vi "p2.vi"() -> ()   [LabVIEW 2021, in "d18.lvlib"]
uses:
  d18.lvlib
  <vilib>/Math Plots/3D Math Plots/3D Scatter/3D Scatter XCtrl/3D Scatter.xctl
  <vilib>/Math Plots/3D Math Plots/3D Scatter/3D Scatter Datatype/Public/Plot Helper (Vector).vi
  AOC/AOC.lvlib
  <vilib>/Math Plots/3D Math Plots/3D Scatter/3D Scatter Datatype/3D Scatter Datatype.lvclass
panel:
  out "3D Scatter":refnum<class "3D Plot Datatype.lvclass">[](xcontrol)
  in  "Example":string="2,2,2\n1,2,2\n3,2,2\n2,1,2\n2,3,2\n2,2,1\n2,2,3\n2,2,4\n2,2,6\n1,2,5\n3,2,5\n2,1,5\n2,3,5"
  in  "Example":bool=TRUE
  out "Answer":i64
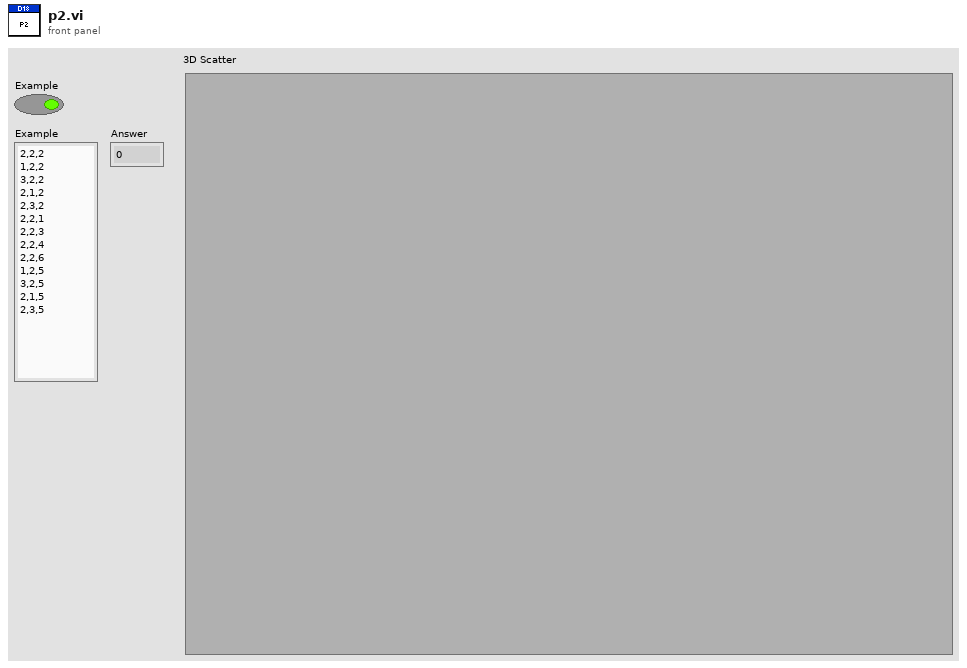
[diagram p1: front panel]
types:
  T1 = cluster{"point":cluster{i64, i64, i64}, "Response Notifier":refnum<notifier>}
  T2 = cluster{cluster{"Point to Set":cluster{i64, i64, i64}, "Internal?":bool}, "notifier out":refnum<notifier>}
  T3 = map{cluster{i64, i64, i64}, cluster{"Set?":bool, "Internal?":bool}}
  T4 = cluster{"key not found?":bool, cluster{"Set?":bool, "Internal?":bool}}
  T5 = cluster{"Point to Set":cluster{i64, i64, i64}, "Internal?":bool}
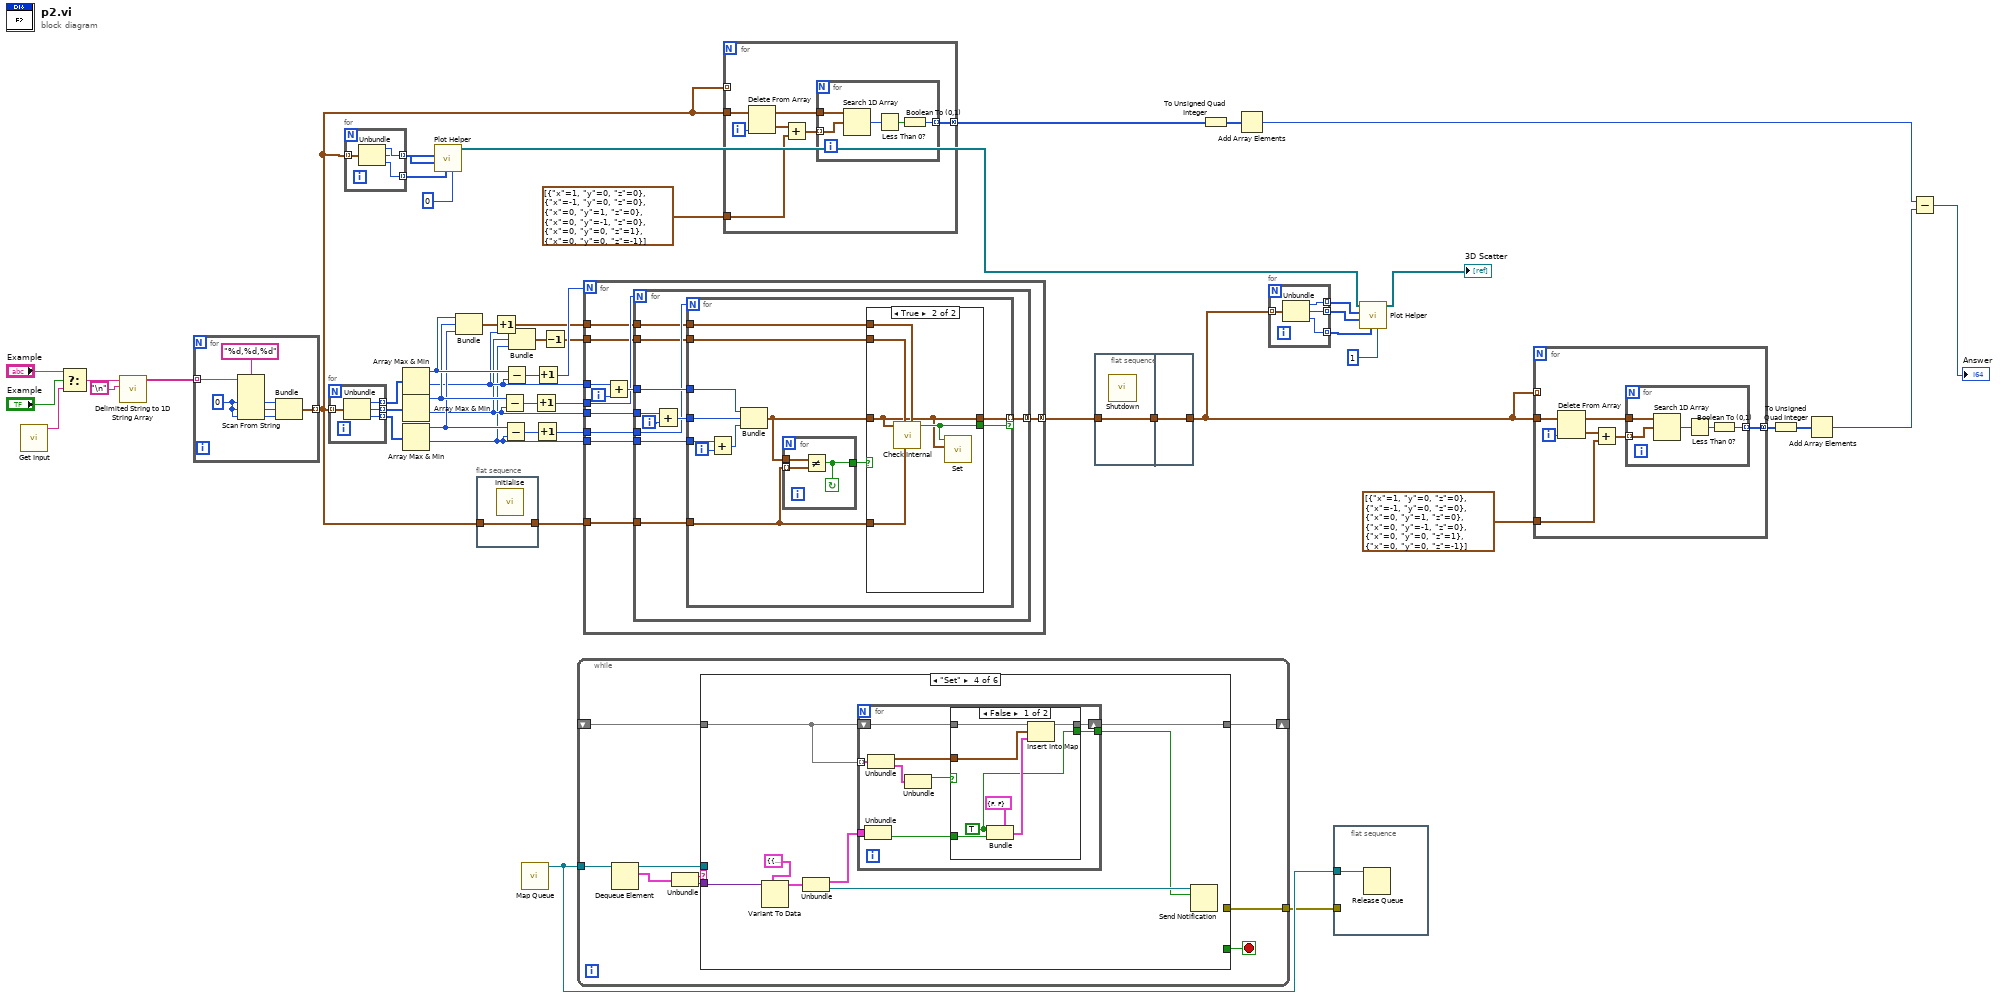
[diagram p0: block diagram]
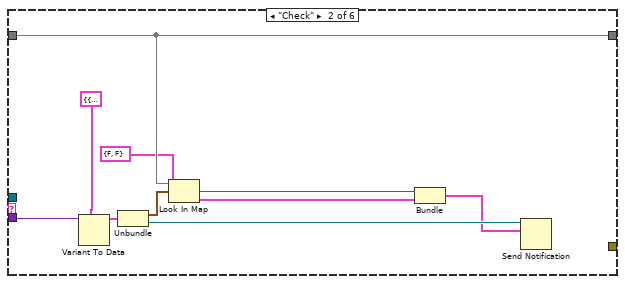
[diagram p3: hidden frame]
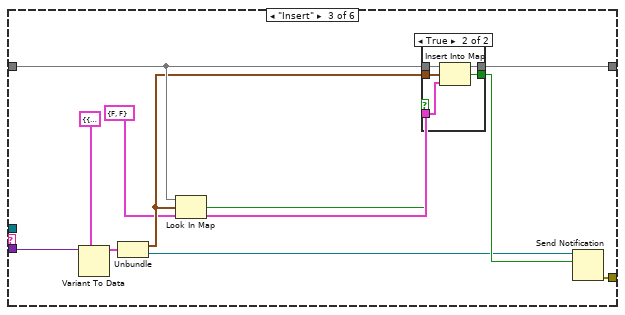
[diagram p4: hidden frame]
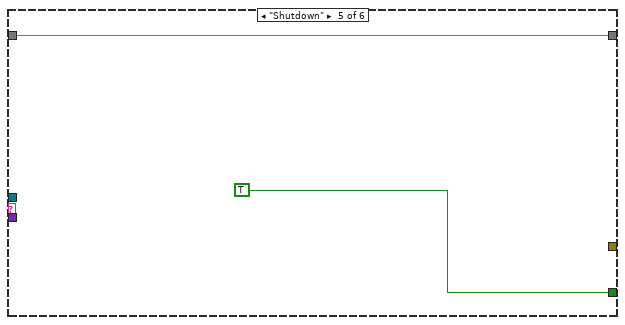
[diagram p7: hidden frame]
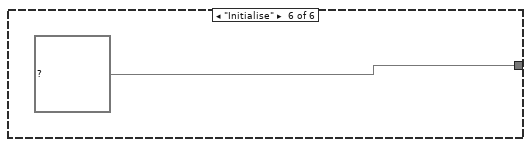
[diagram p8: hidden frame]
diagram:
  n1 = call "Get Input.vi"() -> ("Input"=w51:string)  [unwired: 11 in]
  n2 = Select(t="Example", s="Example", f=w51) -> (s? t:f=w50:string)
  n3 = call <vilib>:"Delimited String to 1D String Array.vi"("delimiter"="\n", "delimited string"=w50) -> ("string array"=w46:string[])  [unwired: 9 in]
  n4 = for {
    tunnel: w46 -> [w58] mode=indexing
    tunnel: [w52] -> w14 mode=indexing
    w56 = i64 0
    n5 = Scan From String(format string="%d,%d,%d", input string=w58, default 1=w56, default 2=w56, default 3=w56) -> (output 1=w55:i64, output 2=w54:i64, output 3=w53:i64)  [unwired: 2 in, 3 out]
    n6 = Bundle(w55, w54, w53) -> (w52:cluster{i64, i64, i64})  [unwired: 1 in]
  }
  n7 = for {
    tunnel: w14 -> [w62] mode=indexing
    tunnel: [w61] -> w45 mode=indexing
    tunnel: [w60] -> w44 mode=indexing
    tunnel: [w59] -> w43 mode=indexing
    n8 = Unbundle(w62) -> (w61:i64, w60:i64, w59:i64)
  }
  n9 = for {
    tunnel: w14 -> [w66] mode=indexing
    tunnel: [w65] -> w13 mode=indexing
    tunnel: [w64] -> w12 mode=indexing
    tunnel: [w63] -> w11 mode=indexing
    n10 = Unbundle(w66) -> (w65:i64, w64:i64, w63:i64)
  }
  n11 = Array Max & Min(array=w45) -> (max value=w36:i64, min value=w33:i64)  [unwired: 2 out]
  n12 = Array Max & Min(array=w44) -> (max value=w35:i64, min value=w32:i64)  [unwired: 2 out]
  n13 = Array Max & Min(array=w43) -> (max value=w34:i64, min value=w31:i64)  [unwired: 2 out]
  n14 = call-poly <vilib>:"Plot Helper.vi"("Plot ID"=0, "z vector"=w11, "y vector"=w12, "x vector"=w13) -> ("3D Plot lvclass Array out"=w9:refnum<class "3D Plot Datatype.lvclass">[])  [unwired: 2 in, 5 out]
  n15 = Bundle(w36, w35, w34) -> (w30:cluster{i64, i64, i64})  [unwired: 1 in]
  n16 = flat-sequence {
    tunnel: w14 -> [w67]
    tunnel: [w67] -> w18
    frame #0 {
      n17 = call "Initialise.vi"() -> ()  [unwired: 12 in]
    }
  }
  n18 = Increment(x=w30) -> (x+1=w2:cluster{i64, i64, i64})
  n19 = Subtract(x=w35, y=w32) -> (x-y=w41:i64)
  n20 = Subtract(x=w34, y=w31) -> (x-y=w39:i64)
  n21 = Subtract(x=w36, y=w33) -> (x-y=w42:i64)
  n22 = Bundle(w33, w32, w31) -> (w29:cluster{i64, i64, i64})  [unwired: 1 in]
  n23 = call "Map Queue.vi"() -> ("Queue out"=w16:refnum<queue>)  [unwired: 11 in]
  n24 = Increment(x=w41) -> (x+1=w40:i64)
  n25 = Increment(x=w39) -> (x+1=w38:i64)
  n26 = Increment(x=w42) -> (x+1=w37:i64)
  n27 = Decrement(x=w29) -> (x-1=w1:cluster{i64, i64, i64})
  n28 = while {
    tunnel: w16 -> [w76]
    shift-right: [w71] -> _
    shift-left: _ -> [w70]
    tunnel: [w68] -> w15
    stop <- w69 stop-if-true
    n29 = Dequeue Element(queue=w76) -> (queue out=w75:refnum<queue>, element=w74:cluster{"Instruction":string, "Data":variant})  [unwired: 2 in, 2 out]
    n30 = Unbundle(w74) -> ("Instruction"=w73:string, "Data"=w72:variant)
    n31 = case shown="\"Set\"" w73 {
      tunnel: w75 -> [_ _ _ _ _ _]
      tunnel: w72 -> [_ w87 w99 w113 _ _]
      tunnel: [w77 w86 w97 w111 w133 T3 {} ("map in")] -> w71
      tunnel: w70 -> [w77 w86 w95 w106 w133 _]
      tunnel: [_ _ _ _ TRUE _] -> w69
      tunnel: [_ _ w88 _ _ _] -> w68
      frame Default {
      }
      frame "Check" {
        n32 = Variant To Data(type=T1 {"point"={0, 0, 0}, "Response Notifier"=refnum}, Variant=w87) -> (data=w85:T1)  [unwired: 1 in, 1 out]
        n33 = Unbundle(w85) -> ("point"=w84:cluster{i64, i64, i64}, "Response Notifier"=w83:refnum<notifier>)
        n34 = Look In Map(map=w86, key=w84, default value=cluster{"Set?":bool, "Internal?":bool} {"Set?"=FALSE, "Internal?"=FALSE}) -> (key not found?=w82:bool, value=w81:cluster{"Set?":bool, "Internal?":bool})
        n35 = Bundle("key not found?"=w82, w81) -> (w80:T4)  [unwired: 1 in]
        n36 = Send Notification(notification=w80, notifier=w83) -> ()  [unwired: 1 in, 2 out]
      }
      frame "Insert" {
        n37 = Variant To Data(type=T1 {"point"={0, 0, 0}, "Response Notifier"=refnum}, Variant=w99) -> (data=w98:T1)  [unwired: 1 in, 1 out]
        n38 = Unbundle(w98) -> ("point"=w94:cluster{i64, i64, i64}, "Response Notifier"=w89:refnum<notifier>)
        n39 = Look In Map(map=w95, key=w94, default value=cluster{"Set?":bool, "Internal?":bool} {"Set?"=FALSE, "Internal?"=FALSE}) -> (key not found?=w91:bool, value=w93:cluster{"Set?":bool, "Internal?":bool})
        n40 = case shown="True" w91 {
          tunnel: [w100 w105] -> w97
          tunnel: [_ w104] -> w96
          tunnel: w95 -> [w100 w103]
          tunnel: w94 -> [_ w102]
          tunnel: w93 -> [_ w101]
          frame False {
          }
          frame True {
            n41 = Insert Into Map(map in=w103, key=w102, value=w101) -> (map out=w105:T3, key already included?=w104:bool)  [unwired: 1 out]
          }
        }
        n42 = Send Notification(notification=w96, notifier=w89) -> (error out=w88:errorcluster)  [unwired: 1 in, 1 out]
      }
      frame "Set" {
        n43 = Variant To Data(type=T2 {{"Point to Set"={0, 0, 0}, "Internal?"=FALSE}, "notifier out"=refnum} ("output cluster"), Variant=w113) -> (data=w112:T2)  [unwired: 1 in, 1 out]
        n44 = Unbundle(w112) -> (w109:T5, "notifier out"=w108:refnum<notifier>)
        n45 = for {
          tunnel: w109 -> [w120]
          tunnel: [w119] -> w107
          shift-right: [w122] -> w111
          shift-left: w106 -> [w121]
          tunnel: w106 -> [w117] mode=indexing
          n46 = Unbundle(w120) -> ("Internal?"=w118:bool)  [unwired: 1 out]
          n47 = Unbundle(w117) -> ("point"=w116:cluster{i64, i64, i64}, "info"=w115:cluster{"Set?":bool, "Internal?":bool})
          n48 = Unbundle(w115) -> ("Set?"=w114:bool)  [unwired: 1 out]
          n49 = case shown="False" w114 {
            tunnel: [w129 w131] -> w122
            tunnel: w121 -> [w128 w131]
            tunnel: [w123 w130] -> w119
            tunnel: w118 -> [w124 w130]
            tunnel: w116 -> [w125 _]
            frame False {
              w123 = TRUE ("Set?")
              n50 = Bundle(cluster=cluster{"Set?":bool, "Internal?":bool} {"Set?"=FALSE, "Internal?"=FALSE} ("value"), "Set?"=w123, "Internal?"=w124) -> (w127:cluster{"Set?":bool, "Internal?":bool})
              n51 = Insert Into Map(map in=w128, key=w125, value=w127) -> (map out=w129:T3)  [unwired: 2 out]
            }
            frame True {
            }
          }
        }
        n52 = Send Notification(notification=w107, notifier=w108) -> ()  [unwired: 1 in, 2 out]
      }
      frame "Shutdown" {
      }
      frame "Initialise" {
      }
    }
  }
  n53 = for {
    N: w37 -> [_]
    tunnel: w33 -> [w145]
    tunnel: w40 -> [w142]
    tunnel: w32 -> [w141]
    tunnel: w38 -> [w140]
    tunnel: w31 -> [w139]
    tunnel: w18 -> [w138]
    tunnel: w2 -> [w137]
    tunnel: w1 -> [w136]
    tunnel: [w135] -> w28 mode=concatenating
    i -> [w144]
    n54 = Add(x=w145, y=w144) -> (x+y=w143:i64)
    n55 = for {
      N: w142 -> [_]
      tunnel: w143 -> [w153]
      tunnel: w141 -> [w155]
      tunnel: w140 -> [w151]
      tunnel: w139 -> [w150]
      tunnel: w138 -> [w149]
      tunnel: w137 -> [w148]
      tunnel: w136 -> [w147]
      tunnel: [w146] -> w135 mode=concatenating
      i -> [w154]
      n56 = Add(x=w155, y=w154) -> (x+y=w152:i64)
      n57 = for {
        N: w151 -> [_]
        tunnel: w153 -> [w165]
        tunnel: w152 -> [w164]
        tunnel: w150 -> [w167]
        tunnel: w149 -> [w156]
        tunnel: w148 -> [w162]
        tunnel: w147 -> [w161]
        tunnel: [w157] -> w146 mode=indexing if=w160
        i -> [w166]
        n58 = Add(x=w167, y=w166) -> (x+y=w163:i64)
        n59 = Bundle(w165, w164, w163) -> (w159:cluster{i64, i64, i64})  [unwired: 1 in]
        n60 = for {
          tunnel: w159 -> [w176]
          tunnel: w156 -> [w175] mode=indexing
          tunnel: [w174] -> w158
          stop <- w174 continue-if-true
          n61 = Not Equal?(x=w176, y=w175) -> (x != y?=w174:bool)
        }
        n62 = case shown="True" w158 {
          tunnel: w162 -> [_ w173]
          tunnel: w161 -> [_ w172]
          tunnel: [_ w170] -> w160
          tunnel: w159 -> [w168 w169]
          tunnel: w156 -> [_ w171]
          tunnel: [w168 w169] -> w157
          frame False {
          }
          frame True {
            n63 = call "Check Internal.vi"("Max Range"=w173, "Points"=w171, "Min Range"=w172, "Point to Check"=w169) -> ("Internal?"=w170:bool)  [unwired: 7 in]
            n64 = call "Set.vi"("Point to Set"=w169, "Internal?"=w170) -> ()  [unwired: 9 in, 1 out]
          }
        }
      }
    }
  }
  n65 = for {
    tunnel: w14 -> [_] mode=indexing
    tunnel: w14 -> [w183]
    tunnel: cluster{"x":i64, "y":i64, "z":i64}[] [{"x"=1, "y"=0, "z"=0}, {"x"=-1, "y"=0, "z"=0}, {"x"=0, "y"=1, "z"=0}, {"x"=0, "y"=-1, "z"=0}, {"x"=0, "y"=0, "z"=1}, {"x"=0, "y"=0, "z"=-1}] -> [w180]
    tunnel: [w177] -> w23 mode=concatenating
    i -> [w182]
    n66 = Delete From Array(array=w183, index=w182) -> (deleted portion=w181:cluster{i64, i64, i64}, array with subset deleted=w179:cluster{i64, i64, i64}[])  [unwired: 1 in]
    n67 = Add(x=w181, y=w180) -> (x+y=w178:cluster{i64, i64, i64}[])
    n68 = for {
      tunnel: w179 -> [w188]
      tunnel: w178 -> [w187] mode=indexing
      tunnel: [w184] -> w177 mode=indexing
      n69 = Search 1D Array(1D array=w188, element=w187) -> (index of element=w186:i32)  [unwired: 1 in]
      n70 = Less Than 0?(x=w186) -> (x < 0?=w185:bool)
      n71 = Boolean To (0,1)(Boolean=w185) -> (0, 1=w184:i16)
    }
  }
  n72 = flat-sequence {
    tunnel: w28 -> [w189]
    tunnel: [w189] -> w17
    tunnel: [w190] -> w7
    tunnel: w17 -> [w190]
    frame #0 {
      n73 = call "Shutdown.vi"() -> ()  [unwired: 12 in]
    }
    frame #1 {
    }
  }
  n74 = To Unsigned Quad Integer(1:w23) -> (0:w22:u64[])
  n75 = Add Array Elements(numeric array=w22) -> (sum=w21:u64)
  n76 = for {
    tunnel: w7 -> [w194] mode=indexing
    tunnel: [w193] -> w6 mode=indexing
    tunnel: [w192] -> w5 mode=indexing
    tunnel: [w191] -> w4 mode=indexing
    n77 = Unbundle(w194) -> (w193:i64, w192:i64, w191:i64)
  }
  n78 = flat-sequence {
    tunnel: w16 -> [w195]
    tunnel: w15 -> [_]
    frame #0 {
      n79 = Release Queue(queue=w195) -> ()  [unwired: 2 in, 3 out]
    }
  }
  n80 = call-poly <vilib>:"Plot Helper.vi"("Plot ID"=1, "z vector"=w4, "y vector"=w5, "x vector"=w6, "3D Plot lvclass Array in"=w9) -> ("3D Plot lvclass Array out"=→"3D Scatter":refnum<class "3D Plot Datatype.lvclass">[])  [unwired: 1 in, 5 out]
  n81 = for {
    tunnel: w7 -> [_] mode=indexing
    tunnel: w7 -> [w202]
    tunnel: cluster{"x":i64, "y":i64, "z":i64}[] [{"x"=1, "y"=0, "z"=0}, {"x"=-1, "y"=0, "z"=0}, {"x"=0, "y"=1, "z"=0}, {"x"=0, "y"=-1, "z"=0}, {"x"=0, "y"=0, "z"=1}, {"x"=0, "y"=0, "z"=-1}] -> [w199]
    tunnel: [w196] -> w26 mode=concatenating
    i -> [w201]
    n82 = Delete From Array(array=w202, index=w201) -> (deleted portion=w200:cluster{i64, i64, i64}, array with subset deleted=w198:cluster{i64, i64, i64}[])  [unwired: 1 in]
    n83 = Add(x=w200, y=w199) -> (x+y=w197:cluster{i64, i64, i64}[])
    n84 = for {
      tunnel: w198 -> [w207]
      tunnel: w197 -> [w206] mode=indexing
      tunnel: [w203] -> w196 mode=indexing
      n85 = Search 1D Array(1D array=w207, element=w206) -> (index of element=w205:i32)  [unwired: 1 in]
      n86 = Less Than 0?(x=w205) -> (x < 0?=w204:bool)
      n87 = Boolean To (0,1)(Boolean=w204) -> (0, 1=w203:i16)
    }
  }
  n88 = To Unsigned Quad Integer(1:w26) -> (0:w25:u64[])
  n89 = Add Array Elements(numeric array=w25) -> (sum=w20:u64)
  n90 = Subtract(x=w21, y=w20) -> (x-y=→"Answer":u64)
